vi "Set Menu for Graph or impedance.vi"(8 "error in (no error)":errorcluster, 10 "String":string, 11 "Menu in":refnum<k9>) -> (3 "Value":enum32{"Graph", "Impedance", "More Options"}(ring))   [LabVIEW 2016, in "CML UI.lvlib"]
uses:
  CML UI.lvlib
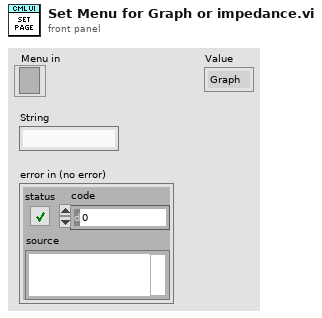
[diagram p1: front panel]
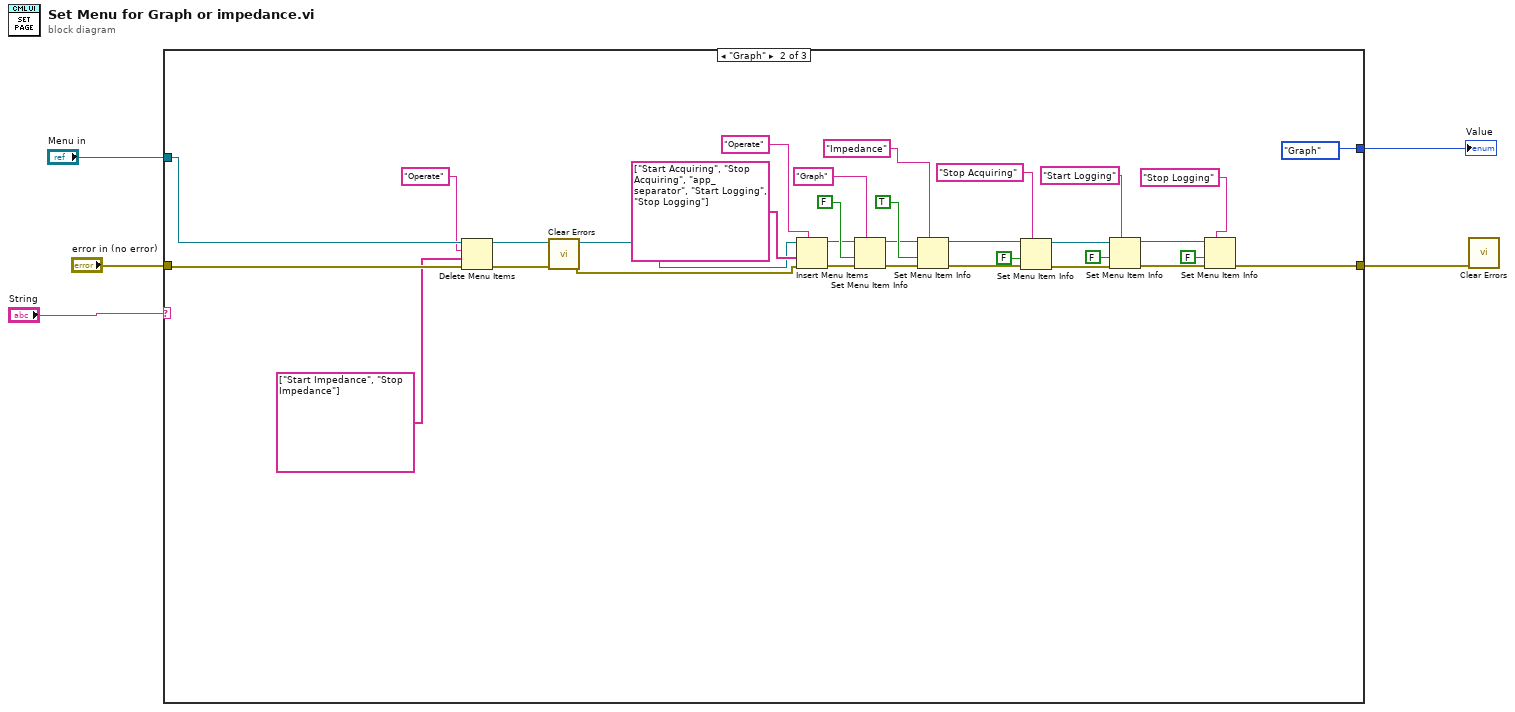
[diagram p0: block diagram]
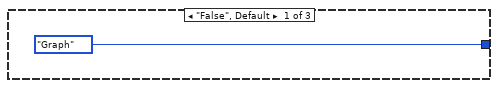
[diagram p2: hidden frame]
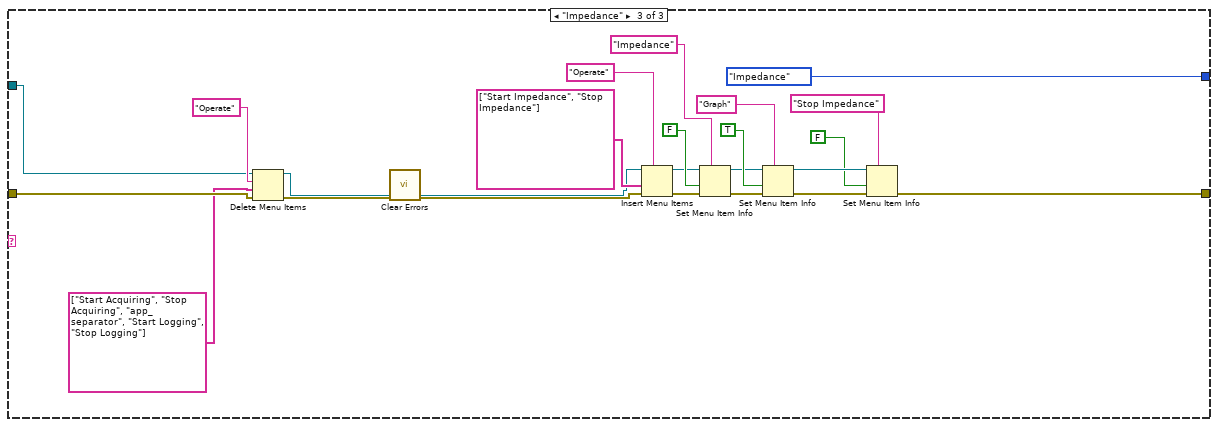
[diagram p3: hidden frame]
diagram:
  n1 = case shown="\"Graph\"" "String" {
    tunnel: [enum32{"Graph", "Impedance", "More Options"}."Graph" ("Value") enum32{"Graph", "Impedance", "More Options"}."Graph" ("Value") enum32{"Graph", "Impedance", "More Options"}."Impedance" ("Value")] -> w2
    tunnel: "Menu in" -> [_ w26 w48]
    tunnel: "error in (no error)" -> [_ w25 w47]
    tunnel: [_ w16 w41] -> w5
    frame "False", Default {
    }
    frame "Graph" {
      n2 = Delete Menu Items(6:w25, 7:string[] ["Start Impedance", "Stop Impedance"] ("L10n_item tags 2"), 8:"Operate" ("L10n_menu tag"), 9:w26) -> (0:w23:errorcluster, 3:w24:refnum<k9>)
      n3 = call <vilib>:"Clear Errors.vi"("error in (no error)"=w23) -> ("error out"=w20:errorcluster)  [unwired: 5 in, 1 out]
      n4 = Insert Menu Items(5:"Operate" ("L10n_menu tag"), 6:w20, 7:string[] ["Start Acquiring", "Stop Acquiring", "app_separator", "Start Logging", "Stop Logging"] ("L10n_item tags 2"), 9:w24) -> (0:w27:errorcluster, 3:w28:refnum<k9>)  [unwired: 2 in, 1 out]
      n5 = Set Menu Item Info(7:"Graph" ("item tag"), 8:w27, 9:FALSE ("enabled"), 11:w28) -> (0:w31:errorcluster, 3:w32:refnum<k9>)  [unwired: 3 in]
      n6 = Set Menu Item Info(7:"Impedance" ("item tag"), 8:w31, 9:TRUE ("enabled"), 11:w32) -> (0:w19:errorcluster, 3:w9:refnum<k9>)  [unwired: 3 in]
      n7 = Set Menu Item Info(7:"Stop Acquiring" ("item tag"), 8:w19, 9:FALSE ("enabled"), 11:w9) -> (0:w18:errorcluster, 3:w8:refnum<k9>)  [unwired: 3 in]
      n8 = Set Menu Item Info(7:"Start Logging" ("item tag"), 8:w18, 9:FALSE ("enabled"), 11:w8) -> (0:w17:errorcluster, 3:w7:refnum<k9>)  [unwired: 3 in]
      n9 = Set Menu Item Info(7:"Stop Logging" ("item tag"), 8:w17, 9:FALSE ("enabled"), 11:w7) -> (0:w16:errorcluster)  [unwired: 3 in, 1 out]
    }
    frame "Impedance" {
      n10 = Delete Menu Items(6:w47, 7:string[] ["Start Acquiring", "Stop Acquiring", "app_separator", "Start Logging", "Stop Logging"] ("L10n_item tags 2"), 8:"Operate" ("L10n_menu tag"), 9:w48) -> (0:w46:errorcluster, 3:w45:refnum<k9>)
      n11 = call <vilib>:"Clear Errors.vi"("error in (no error)"=w46) -> ("error out"=w44:errorcluster)  [unwired: 5 in, 1 out]
      n12 = Insert Menu Items(5:"Operate" ("L10n_menu tag"), 6:w44, 7:string[] ["Start Impedance", "Stop Impedance"] ("L10n_item tags 2"), 9:w45) -> (0:w50:errorcluster, 3:w51:refnum<k9>)  [unwired: 2 in, 1 out]
      n13 = Set Menu Item Info(7:"Impedance" ("item tag"), 8:w50, 9:FALSE ("enabled"), 11:w51) -> (0:w54:errorcluster, 3:w55:refnum<k9>)  [unwired: 3 in]
      n14 = Set Menu Item Info(7:"Graph" ("item tag"), 8:w54, 9:TRUE ("enabled"), 11:w55) -> (0:w42:errorcluster, 3:w40:refnum<k9>)  [unwired: 3 in]
      n15 = Set Menu Item Info(7:"Stop Impedance" ("item tag"), 8:w42, 9:FALSE ("enabled"), 11:w40) -> (0:w41:errorcluster)  [unwired: 3 in, 1 out]
    }
  }
  "Value" <- w2
  n16 = call <vilib>:"Clear Errors.vi"("error in (no error)"=w5) -> ()  [unwired: 5 in, 2 out]
